vi "HackRF_SetGain_RxVGA.vi"(8 "error in (no error)":errorcluster, 10 "VGAGainDb":dbl min=0.0 max=62.0 step=2.0, 11 "HackRF in":T1) -> (0 "error out":errorcluster, 3 "HackRF out":T1)   [LabVIEW 2010]
doc: "baseband (\"vga\", 0 to 62 dB in 2 dB steps)\n\nThe three RX gain controls are at the RF (\"amp\", 0 or 14 dB), IF gain (\"lna\", 0 to 40 dB in 8 dB steps), and baseband (\"vga\", 0 to 62 dB in 2 dB steps) stages."
uses:
  HackRF_Ref.ctl
  C:/Program Files/HackRF/labview/x86/NetHackrf.dll
  NetHackrf.dll
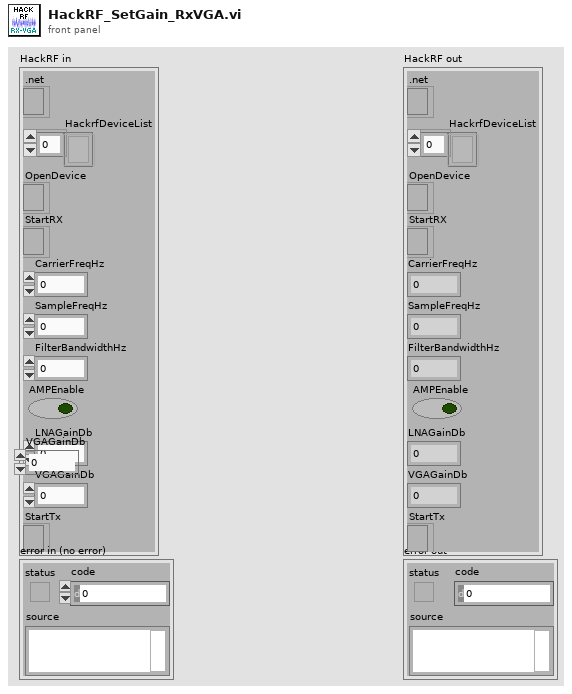
[diagram p1: front panel]
types:
  T1 = typedef "HackRF_Ref.ctl" = cluster{".net":refnum<k24>, "HackrfDeviceList":refnum<k24>[], "OpenDevice":refnum<k24>, "StartRX":refnum<k24>, "CarrierFreqHz":dbl, "SampleFreqHz":dbl, "FilterBandwidthHz":dbl, "AMPEnable":bool, "LNAGainDb":dbl, "VGAGainDb":dbl, "StartTx":refnum<k24>}
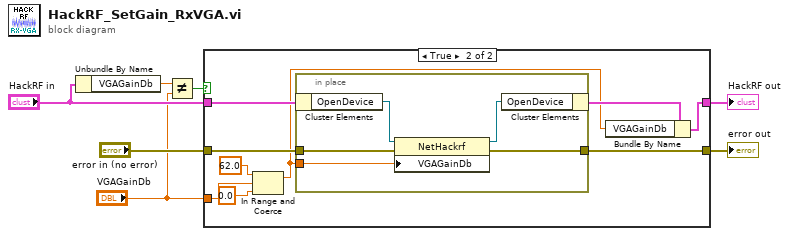
[diagram p0: block diagram]
diagram:
  n1 = Unbundle By Name("HackRF in") -> ("VGAGainDb"=w3:dbl)
  n2 = Not Equal?(x=w3, y="VGAGainDb") -> (x != y?=w1:bool)
  n3 = case shown="True" w1 {
    tunnel: "error in (no error)" -> [w9 w18]
    tunnel: [w9 w17] -> w6
    tunnel: [w8 w14] -> w5
    tunnel: "HackRF in" -> [w8 w16]
    tunnel: "VGAGainDb" -> [_ w13]
    frame False {
    }
    frame True {
      n4 = In Range and Coerce(upper limit=62.0, x=w13, lower limit=0.0) -> (coerced(x)=w12:dbl)  [unwired: 1 out]
      n5 = in-place {
        in-place-border: w18 -> [w21]
        in-place-border: [w20] -> w17
        in-place-border: w12 -> [w19]
        n6 = in-place-cluster #1(w16) -> ("OpenDevice"=w23:refnum<k24>)
        n7 = property class="NetHackrf"(reference=w23, error in=w21, "VGAGainDb"=w19) -> (reference out=w22:refnum<k24>, error out=w20:errorcluster)
        n8 = in-place-cluster #1("OpenDevice"=w22) -> (w15:T1)
      }
      n9 = Bundle By Name(cluster=w15, "VGAGainDb"=w12) -> (w14:T1)
    }
  }
  "error out" <- w6
  "HackRF out" <- w5
